vi "MES_Get PLC Address.vi"(0 "StationName":string, 1 "LineNum":string, 5 "Main":string, 9 "VariableName":string, 11 "error in (no error)":errorcluster, 12 "Alarm":bool=TRUE) -> (3 "IPList":string[](array[string]), 4 "Value":T1, 10 "Array":bool[](array[boolean]), 13 "PLC DB DBB2List":string[](array[string]), 14 "PLC DB DBB1List":string[](array[string]), 15 "error out":errorcluster)   [LabVIEW 2021, in "SQLite.lvclass"]
doc: "读取MES与PLC通讯的IP地址，DB块，DBB地址，format\n# 2020-5-13 13:25:16\n# daikinyi\n蒋松\njiangsong@outlook.com"
uses:
  SQLite.lvclass
  Control/PLCAddress value Type.ctl
  SQLiteFileName.ctl
  TabelFullName.ctl
  <userlib>/LabSQL/LabSQL.lvlib
  <userlib>/sushu/sushu.lvlib
panel:
  out "number (0 to 1)":dbl
  out "Select SQL CMD":string
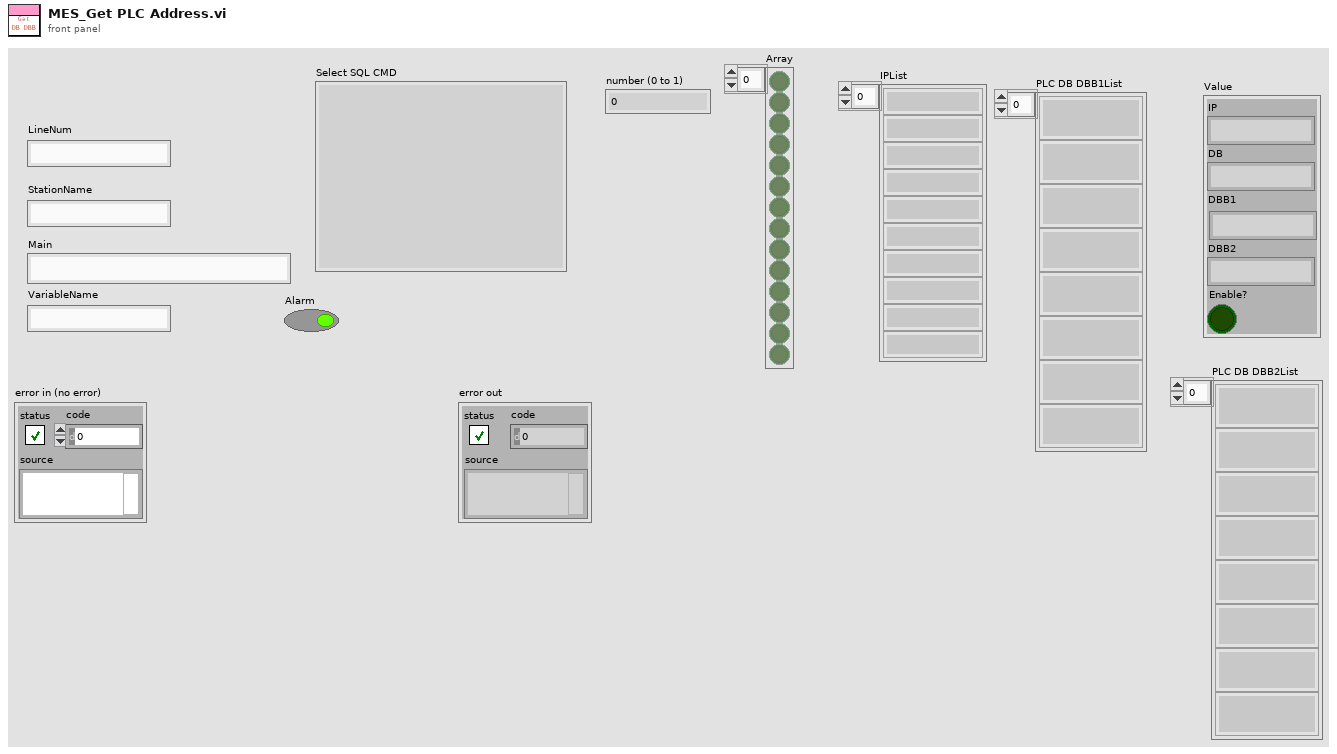
[diagram p1: front panel]
types:
  T1 = typedef "SQLite.lvclass/PLCAddress value Type.ctl" = cluster{"IP":string, "DB":string, "DBB1":string, "DBB2":string, "Enable?":bool}
  T2 = enum16{"Initialize", "Read", "Write", "UnInitialize"}
  T3 = typedef "SQLite.lvclass/TabelFullName.ctl" = string
  T4 = typedef "SQLite.lvclass/SQLiteFileName.ctl" = string
  T5 = cluster{"Current VI Reference":refnum<vi>, "Close Panel on Exit?":bool}
  T6 = cluster{"Core":cluster{"Current VI Reference":refnum<vi>, "Close Panel on Exit?":bool}, "VI Name":string}
  T7 = enum16{"Other", "SQL2008", "SQLite", "Access", "MySQL"}
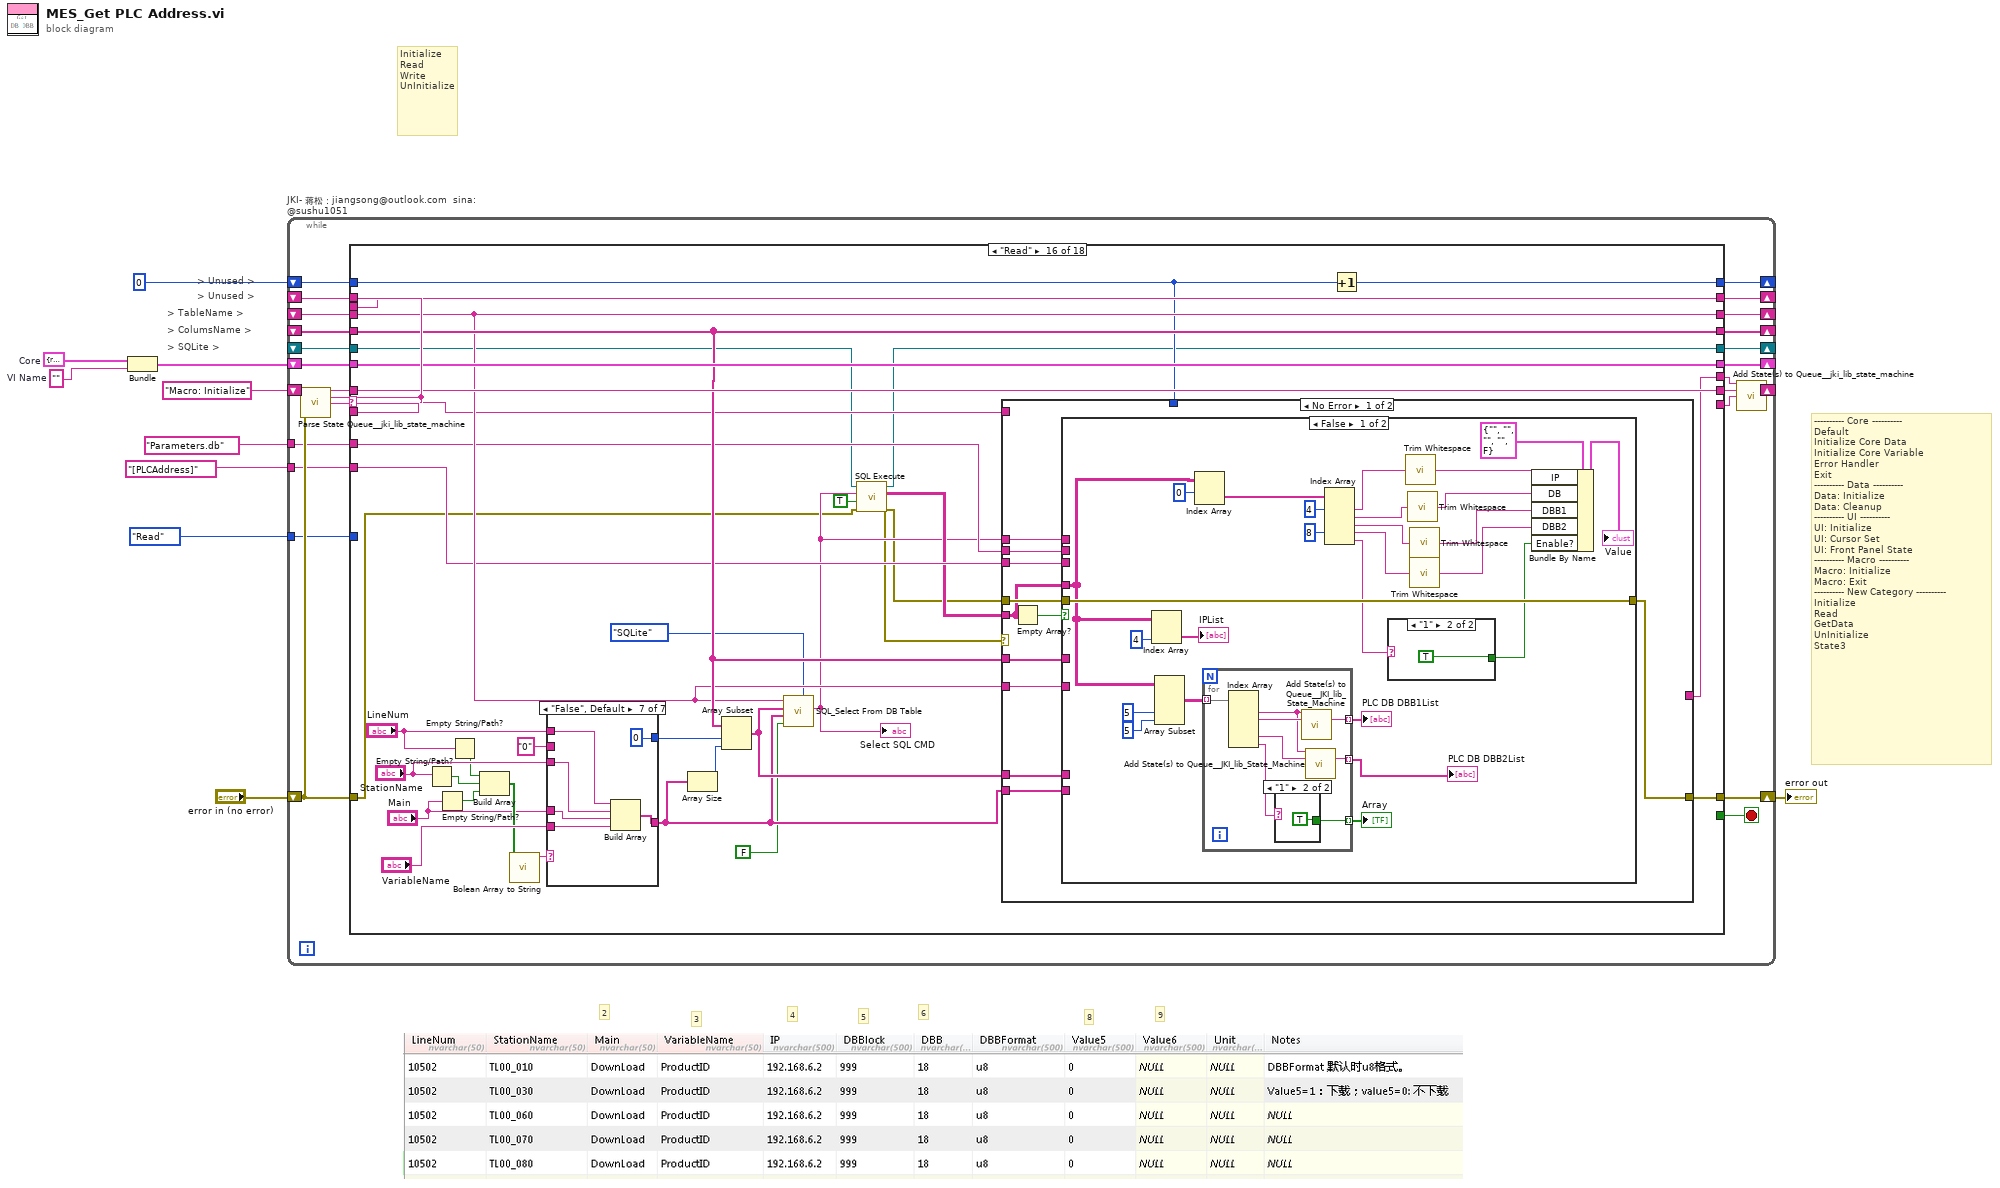
[diagram p0: block diagram]
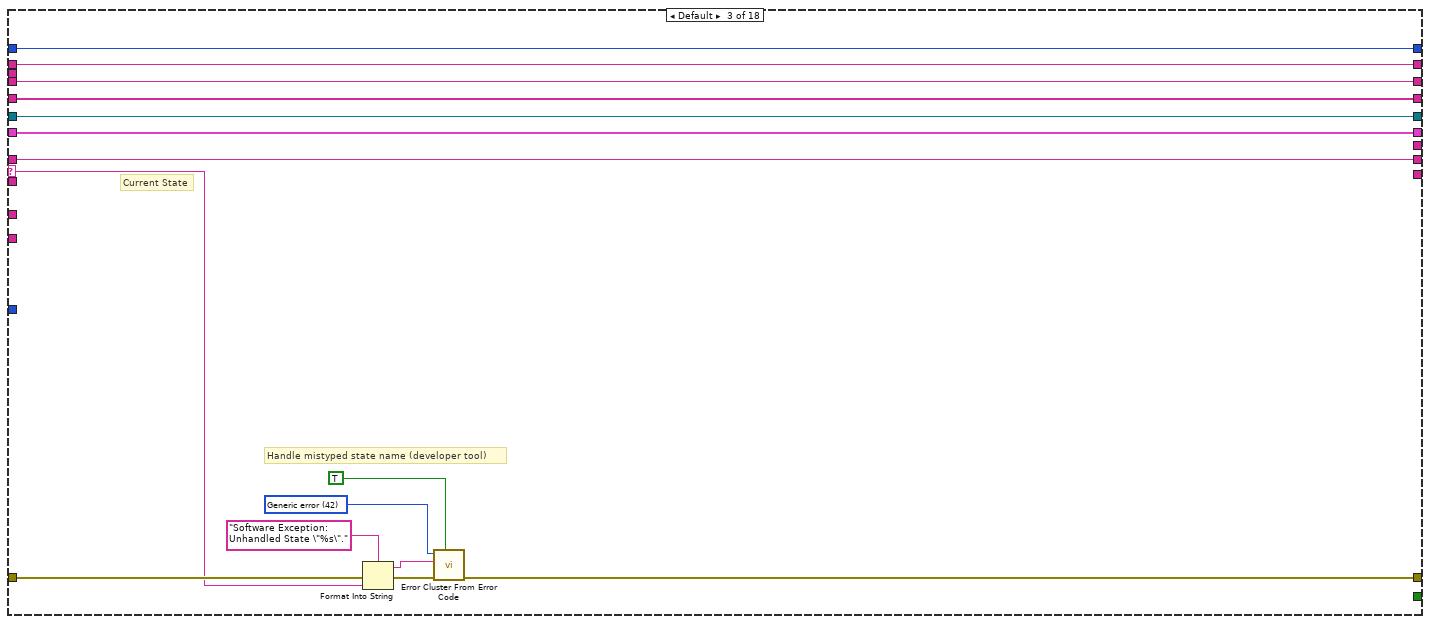
[diagram p4: hidden frame]
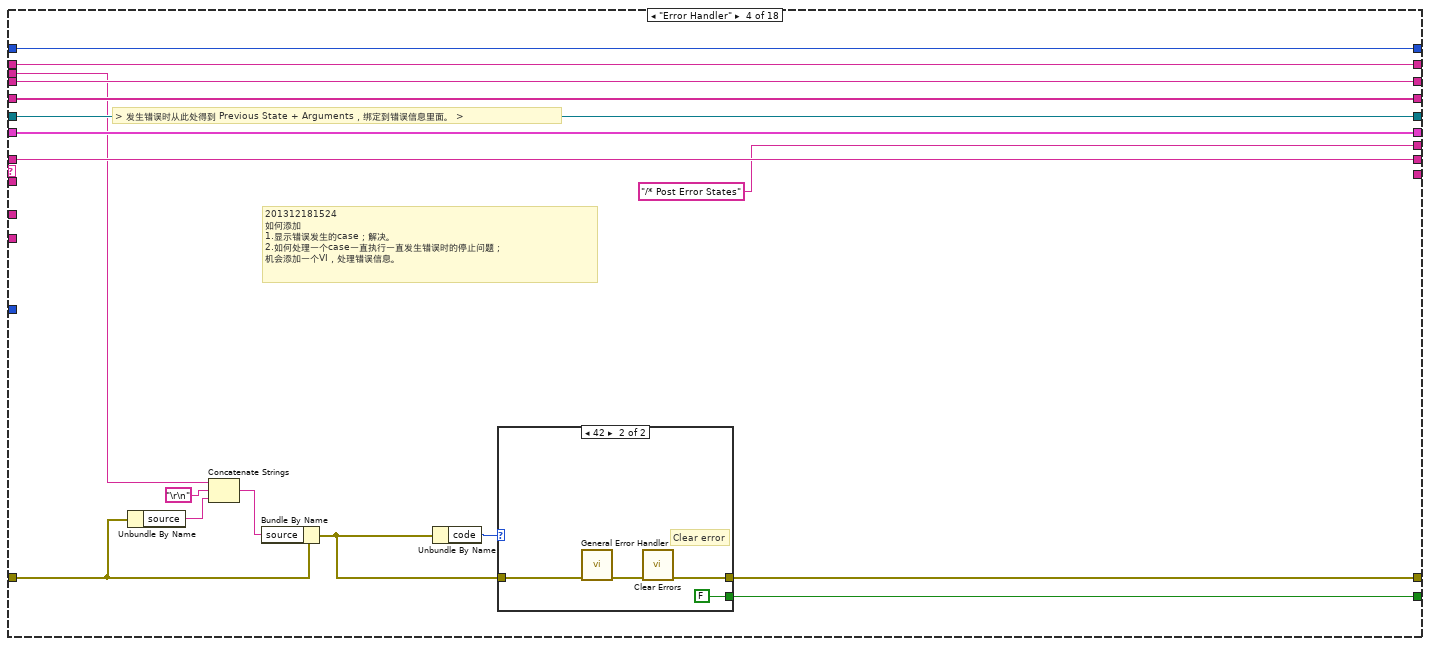
[diagram p5: hidden frame]
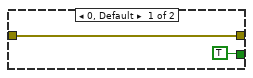
[diagram p6: hidden frame]
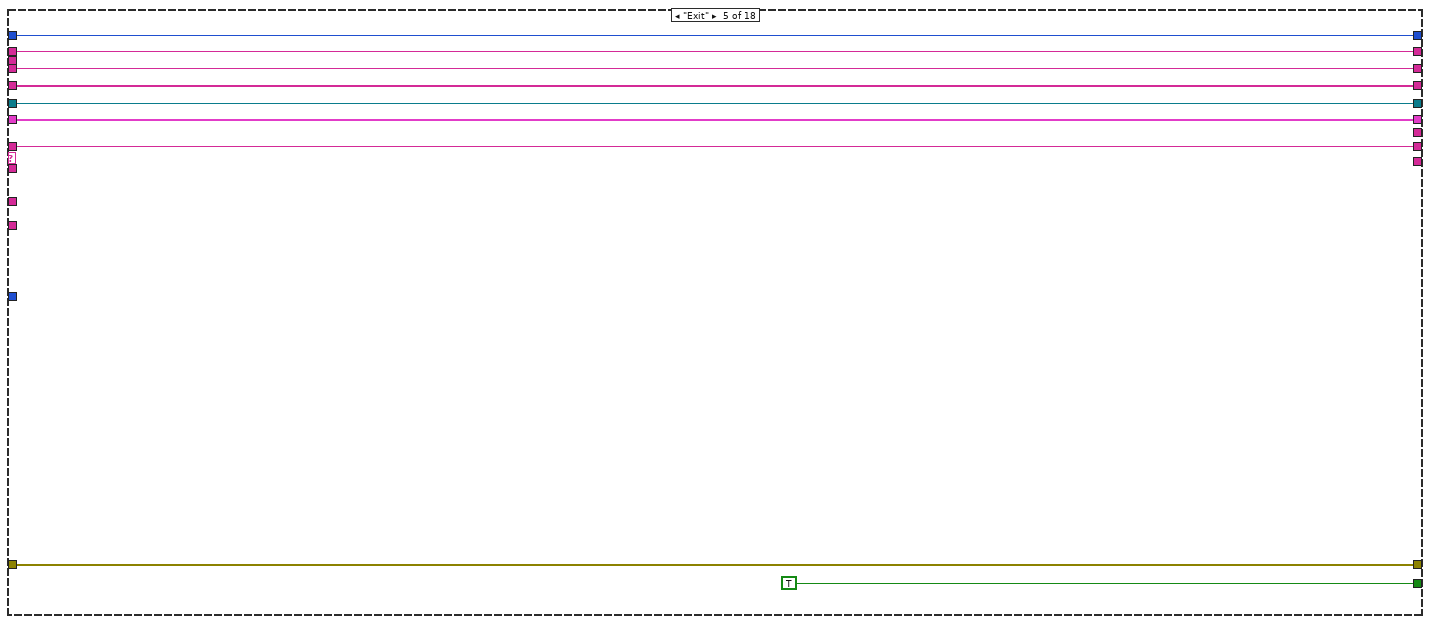
[diagram p7: hidden frame]
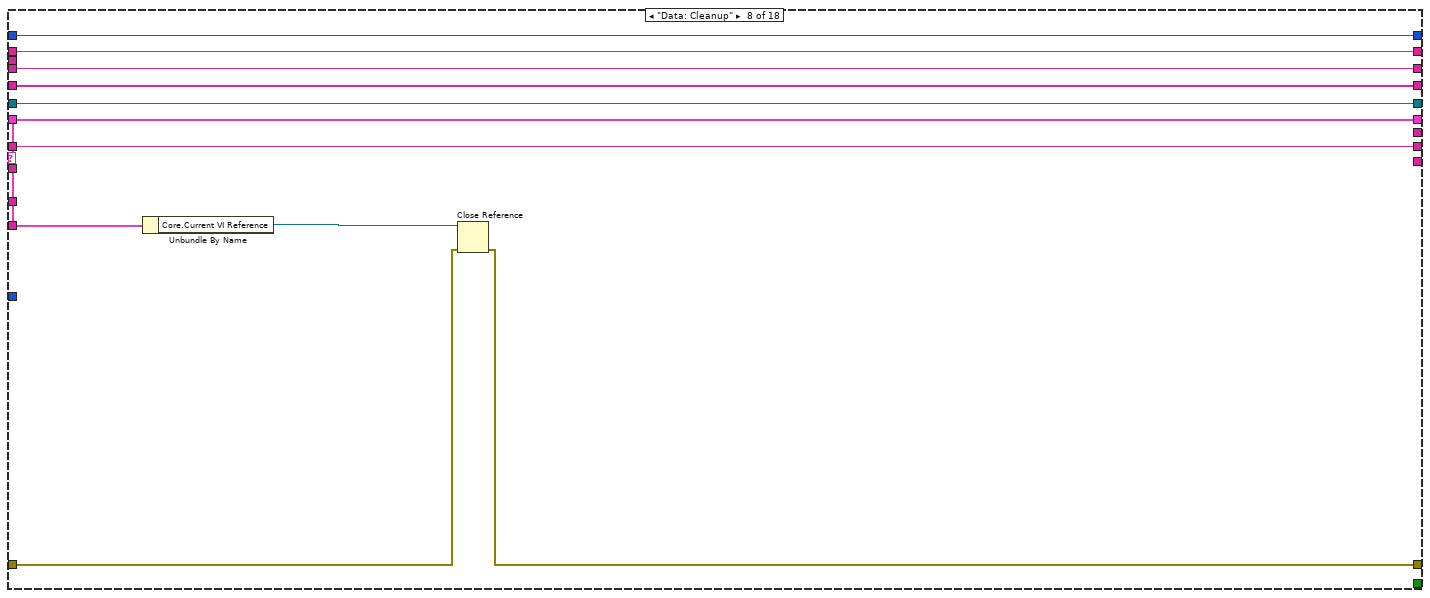
[diagram p10: hidden frame]
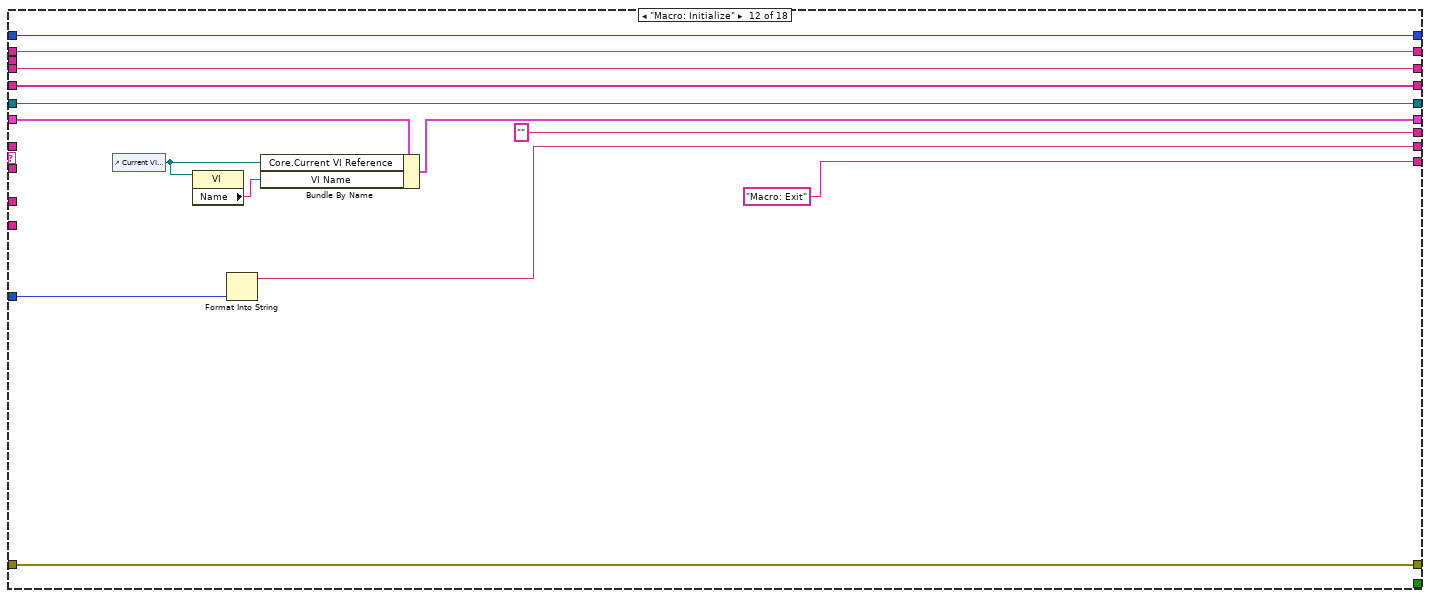
[diagram p14: hidden frame]
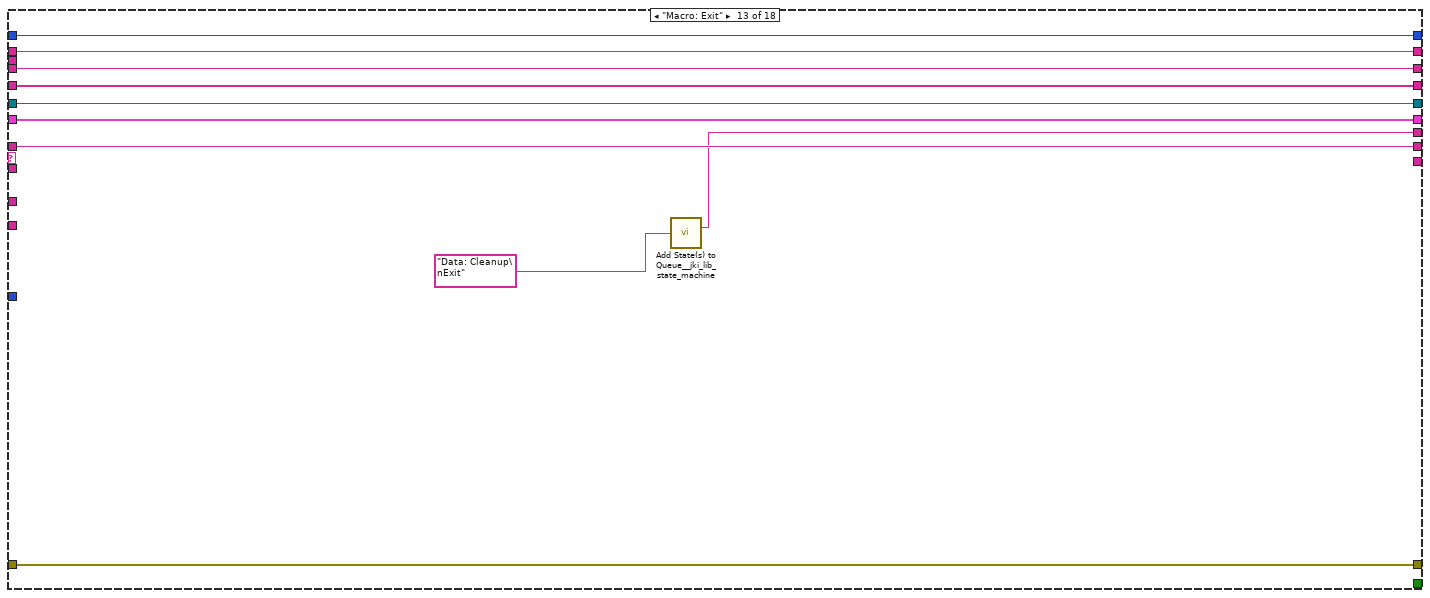
[diagram p15: hidden frame]
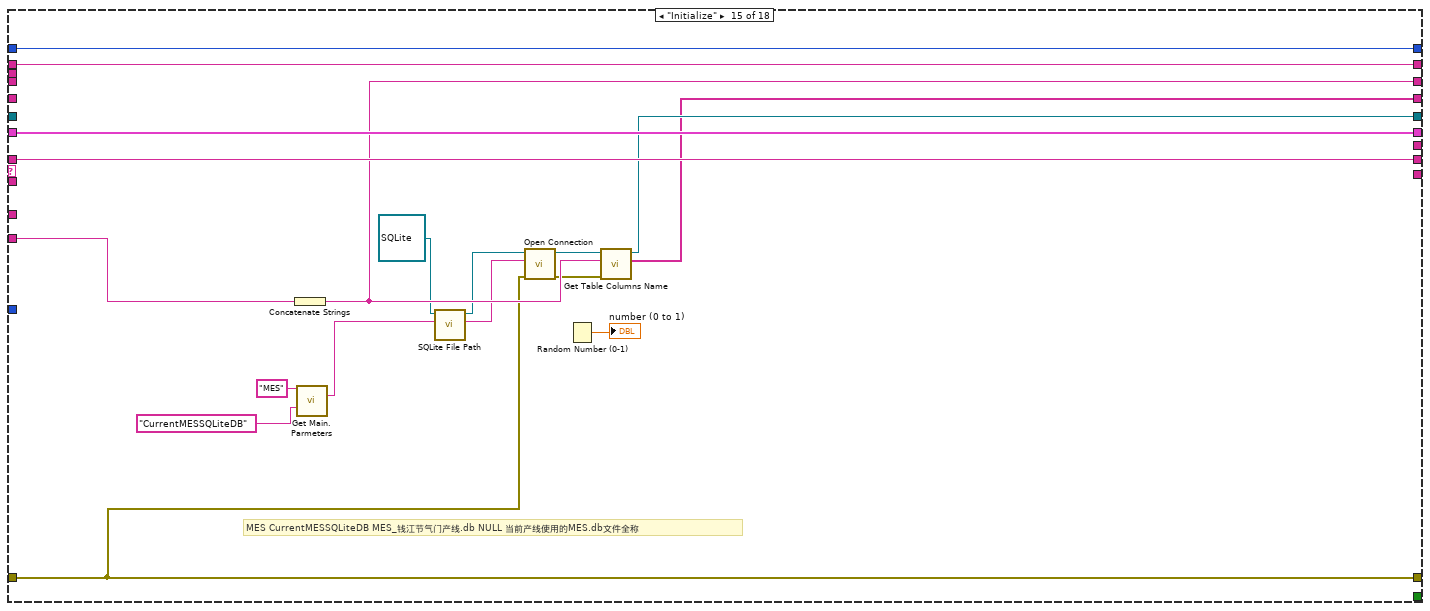
[diagram p17: hidden frame]
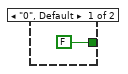
[diagram p18: hidden frame]
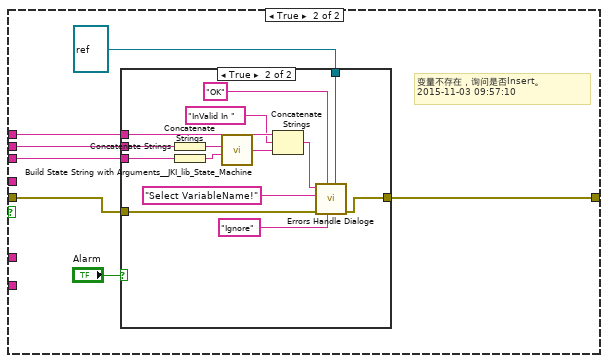
[diagram p20: hidden frame]
diagram:
  w10 = ""  # VI Name
  w9 = T5 {"Current VI Reference"=refnum, "Close Panel on Exit?"=FALSE}  # Core
  # "9"
  # "8"
  # "2"
  # "6"
  # "5"
  # "4"
  # "3"
  # "Initialize\nRead\nWrite\nUnInitialize"
  # "> Unused >"
  # "> SQLite >"
  # "> ColumsName >"
  # "> TableName >"
  # "> Unused >"
  # "---------- Core ----------\nDefault\nInitialize Core Data\nInitialize Core Variable\nError Handler\nExit\n---------- Data ----------\nData: Initialize\nData: Cleanup\n---------- UI ----------\nUI: Initialize\nUI: Cursor Set\nUI: Front Panel State\n---------- Macro ----------\nMacro: Initialize\nMacro: Exit\n---------- New Category ----------\nInitialize\nRead\nGetData\nUnInitialize\nState3"
  n1 = Bundle("Core"=w9, "VI Name"=w10) -> (w8:T6)  [unwired: 1 in]
  n2 = while "JKI- 蒋松：jiangsong@outlook.com  sina: @sushu1051" {
    shift-right: [w34] -> w3
    shift-left: "error in (no error)" -> [w32]
    shift-right: [w22] -> _
    shift-left: "Macro: Initialize" -> [w23]
    shift-right: [w29] -> _
    shift-left: _ -> [w31]
    shift-right: [w30] -> _
    shift-left: _ -> [w11]
    shift-right: [w24] -> _
    shift-left: w8 -> [w27]
    shift-right: [w25] -> _
    shift-left: _ -> [w18]
    shift-right: [w26] -> _
    shift-left: _ -> [w28]
    shift-right: [w17] -> _
    shift-left: 0 -> [w16]
    tunnel: T2."Read" ("CMD") -> [w15]
    tunnel: T4 "Parameters.db" ("SQLiteFileName") -> [w14]
    tunnel: T3 "[PLCAddress]" ("TabelFullName") -> [w13]
    stop <- w33 stop-if-true
    n3 = call <vilib>:"Parse State Queue__jki_lib_state_machine.vi"("State Queue"=w23, "Error In (no error)"=w32) -> ("Remaining States"=w36:string, "Current State"=w12:string, "Arguments"=w35:string)  [unwired: 10 in, 1 out]
    n4 = case shown="\"Read\"" w12 {
      selector: w12 -> [_ _ w55 _ _ _ _ _ _ _ _ _ _ _ _ w220 _ _]
      tunnel: w36 -> [w44 w46 w54 w76 w92 w101 w110 w117 w127 w135 w143 _ w166 w175 w199 w234 w361 w371]
      tunnel: w35 -> [_ _ _ _ _ _ _ _ _ _ _ _ _ _ _ _ _ _]
      tunnel: [w43 w52 w56 w70 w94 w103 w112 w119 w129 w137 w145 w160 w170 w178 w189 w221 w354 w362] -> w34
      tunnel: w32 -> [w43 w52 w57 w80 w94 w103 w112 w120 w129 w137 w145 w160 w170 w178 w189 w213 w354 w363]
      tunnel: [w44 w46 w54 w76 w92 w101 w110 w117 w127 w135 w143 w151 w166 w175 w199 w234 w361 w371] -> w21
      tunnel: [_ _ _ w69 TRUE _ _ _ _ _ _ _ _ _ _ _ _ _] -> w33
      tunnel: w12 -> [w42 w51 w67 w84 w99 w107 w115 w125 w133 w141 w149 w163 w173 w181 w198 w222 w355 w370]
      tunnel: w31 -> [w41 w50 w66 w83 w98 w106 w114 w124 w132 w140 w148 w162 w172 w180 _ w225 w360 w369]
      tunnel: [w42 w51 w67 w84 w99 w107 w115 w125 w133 w141 w149 w163 w173 w181 w198 w222 w355 w370] -> w30
      tunnel: [w41 w50 w66 w83 w98 w106 w114 w124 w132 w140 w148 w162 w172 w180 w191 w225 w360 w369] -> w29
      tunnel: w28 -> [w40 w49 w65 w82 w97 w105 w113 w123 w131 w139 w147 w161 w171 w179 _ w226 w359 w368]
      tunnel: w18 -> [w38 w47 w64 w74 w93 w102 w111 w118 w128 w136 w144 w159 w167 w176 _ w217 w358 w365]
      tunnel: w27 -> [w39 w48 w63 w81 w96 w104 w108 w121 w130 w138 w146 w153 w168 w177 w197 w233 w357 w367]
      tunnel: [w40 w49 w65 w82 w97 w105 w113 w123 w131 w139 w147 w161 w171 w179 w192 w226 w359 w368] -> w26
      tunnel: [w38 w47 w64 w74 w93 w102 w111 w118 w128 w136 w144 w159 w167 w176 w193 w215 w358 w364] -> w25
      tunnel: [w39 w48 w63 w81 w96 w104 w108 w121 w130 w138 w146 w152 w168 w177 w197 w233 w357 w367] -> w24
      tunnel: [_ _ _ "/* Post Error States" _ _ _ _ _ _ _ "" w165 _ _ w219 _ _] -> w20
      tunnel: [_ _ _ _ _ _ _ _ _ _ _ "Macro: Exit" _ _ _ _ _ _] -> w19
      tunnel: w16 -> [w37 w45 w53 w73 w91 w100 w109 w116 w126 w134 w142 w158 w164 w174 w196 w218 w356 w366]
      tunnel: [w37 w45 w53 w73 w91 w100 w109 w116 w126 w134 w142 w158 w164 w174 w196 w232 w356 w366] -> w17
      tunnel: w15 -> [_ _ _ _ _ _ _ _ _ _ _ w150 _ _ _ _ _ _]
      tunnel: w14 -> [_ _ _ _ _ _ _ _ _ _ _ _ _ _ _ w223 _ _]
      tunnel: w13 -> [_ _ _ _ _ _ _ _ _ _ _ _ _ _ w194 w224 _ _]
      tunnel: w11 -> [_ _ _ w68 _ _ _ _ _ _ _ _ _ _ _ _ _ _]
      frame "Idle" {
      }
      frame "---------- Core ----------" {
      }
      frame Default {
        w59 = 42 items=["No error", "Argument error", "Memory is full", "Out of zone", "End of file", "File already open", "Generic file I/O error", "File not found", "File permission error", "Disk is full", "Duplicate path", "Too many files open", "System feature not enabled", "Resource file not found", "Cannot add resource", "Resource not found", "Image not found", "Image memory error", "Pen does not exist", "Config type invalid", "Config token not found", "Config parse error", "Config memory error", "Bad external code format", "Bad external code offset", "External code not present", "Null window", "Destroy window error", "Null menu", "Print aborted", "Bad print record", "Print driver error", "Windows error during printing", "Memory error during printing", "Print dialog error", "Generic print error", "Invalid device refnum", "Device not found", "Device parameter error", "Device unit error", "Cannot open device", "Device call aborted", "Generic error", "Cancelled by user", "Object ID too low", "Object ID too high", "Object not in heap", "Unknown heap", "Unknown object (invalid DefProc)", "Unknown object (DefProc not in table)", "Message out of range", "Invalid (null) method", "Unknown message", "Manager call not supported", "Bad address", "Network operation in progress", "Network operation timed out", "Connection is busy", "Network attribute not supported", "Network error", "Address in use", "System out of memory", "Connection aborted", "Connection refused", "Not connected", "Already connected", "Connection closed", "Initialization error (interapplication manager)", "Bad occurrence", "Wait on unbound occurrence handler", "Occurrence queue overflow", "Datalog type conflict", "Unused", "Unrecognized type (interapplication manager)", "Memory corrupt", "Failed to make temporary DLL", "Old CIN version", "Drag socket not found", "Failed to load drop-object", "Failed to register OLE object", "Failed to release OLE object", "Format specifier type mismatch", "Unknown format specifier", "Too few format specifiers", "Too many format specifiers", "Scan failed", "Newer CIN version", "Error converting to variant", "Runtime menu error", "Password tampered", "Variant attribute not found", "Incompatible variant data type", "Event data is not available", "Event Store is not present", "Occurrence is not found", "Event Queue is not created", "Event info is not available", "Refnum passed is NULL", "Error retrieving Class GUID", "Error retrieving CoClass GUID", "Error retrieving TypeLib GUID.", "Bad built application magic bytes.", "Specific driver is different from the specific driver associated with the Logical Name.", "There is no session opened to the class driver.", "Max Error", "MAX - Error with config objects", "MAX - Error loading configuration", "MAX - Group not supported"]
        # "Current State"
        # "Handle mistyped state name (developer tool)"
        n5 = Format Into String(format string="Software Exception: Unhandled State \"%s\"." ("message"), error in=w57, w55) -> (resulting string=w60:string, error out=w61:errorcluster)  [unwired: 1 in]
        n6 = call <vilib>:"Error Cluster From Error Code.vi"("show call chain? (False)"=TRUE, "error in (no error)"=w61, "error message (\"\")"=w60, "error code (0)"=w59) -> ("error out"=w56:errorcluster)  [unwired: 5 in]
      }
      frame "Error Handler" {
        # "> 发生错误时从此处得到 Previous State + Arguments，绑定到错误信息里面。 >"
        # "201312181524\n如何添加\n1.显示错误发生的case；解决。\n2.如何处理一个case一直执行一直发生错误时的停止问题；\n机会添加一个VI，处理错误信息。"
        # "Clear error"
        n7 = Unbundle By Name(w80) -> ("source"=w78:string)
        n8 = Concatenate Strings(w68, "\r\n", w78) -> (w77:string)
        n9 = Bundle By Name(cluster=w80, "source"=w77) -> (w71:errorcluster)
        n10 = Unbundle By Name(w71) -> ("code"=w72:i32)
        n11 = case shown="42" w72 {
          tunnel: [TRUE FALSE] -> w69
          tunnel: w71 -> [w86 w89]
          tunnel: [w86 w87] -> w70
          frame 0, Default {
          }
          frame 42 {
            n12 = call <vilib>:"General Error Handler.vi"("error in (no error)"=w89) -> ("error out"=w88:errorcluster)  [unwired: 10 in, 4 out]
            n13 = call <vilib>:"Clear Errors.vi"("error in (no error)"=w88) -> ("error out"=w87:errorcluster)  [unwired: 5 in, 1 out]
          }
        }
      }
      frame "Exit" {
      }
      frame "---------- Data ----------" {
      }
      frame "Data: Initialize" {
      }
      frame "Data: Cleanup" {
        n14 = Unbundle By Name(w121) -> ("Core.Current VI Reference"=w122:refnum<vi>)
        n15 = Close Reference(reference=w122, error in (no error)=w120) -> (error out=w119:errorcluster)
      }
      frame "---------- UI ----------" {
      }
      frame "UI: Initialize" {
      }
      frame "---------- Macro ----------" {
      }
      frame "Macro: Initialize" {
        n16 = control-ref of="Current VI Reference"() -> (w154:refnum<vi>)
        n17 = property class="VI"(reference=w154) -> ("Name"=w155:string)  [unwired: 1 in, 2 out]
        n18 = Format Into String(w150) -> (resulting string=w151:string)  [unwired: 3 in, 1 out]
        n19 = Bundle By Name(cluster=w153, "Core.Current VI Reference"=w154, "VI Name"=w155) -> (w152:T6)
      }
      frame "Macro: Exit" {
        n20 = call <vilib>:"Add State(s) to Queue__jki_lib_state_machine.vi"("State(s) at Back (\"\")"="Data: Cleanup\nExit") -> ("States Out"=w165:string)  [unwired: 14 in]
      }
      frame "---------- New Category ----------" {
      }
      frame "Initialize" {
        # "MES\tCurrentMESSQLiteDB\tMES_钱江节气门产线.db\tNULL\t当前产线使用的MES.db文件全称"
        n21 = Concatenate Strings(w194) -> (w191:string)
        n22 = call "Get Main.Parmeters.vi"("Main"="MES", "VariableName"="CurrentMESSQLiteDB" ("Main")) -> ("Value"=w182:string)  [unwired: 6 in, 7 out]
        n23 = call "SQLite File Path.vi"("SQLiteFileName"=w182, "SQLite in"=refnum<class "SQLite.lvclass"> refnum ("SQLite.lvclass")) -> ("string"=w188:string, "SQLite out"=w186:refnum<class "SQLite.lvclass">)  [unwired: 7 in, 1 out]
        n24 = call-dynamic "Open Connection.vi"("error in (no error)"=w189, "ConnectionString"=w188, "HostDB in"=w186) -> ("error out"=w190:errorcluster, "HostDB out"=w195:refnum<class "SQLite.lvclass">)  [unwired: 7 in]
        n25 = Random Number (0-1)() -> (number: 0 to 1=→"number (0 to 1)":dbl)
        n26 = call-dynamic "Get Table Columns Name.vi"("error in (no error)"=w190, "TableName"=w191, "HostDB in"=w195) -> ("Table_ColunmsList"=w192:string[], "HostDB out"=w193:refnum<class "SQLite.lvclass">)  [unwired: 4 in, 3 out]
      }
      frame "Read" {
        n27 = Empty String/Path?(string/path="StationName") -> (empty?=w209:bool)
        n28 = Empty String/Path?(string/path="Main") -> (empty?=w208:bool)
        n29 = Empty String/Path?(string/path="LineNum") -> (empty?=w202:bool)
        n30 = Build Array(w202, w209, w208) -> (w207:bool[])
        n31 = call <userlib>:"Bolean Array to String.vi"("Bolean Array"=w207) -> ("Bolean String"=w206:string)  [unwired: 10 in]
        n32 = case shown="\"False\", Default" w206 {
          tunnel: [w322 w326 w329 w335 w341 w347 w353] -> w229
          tunnel: "Main" -> [w321 w323 _ w332 _ w342 w352]
          tunnel: "VariableName" -> [w320 w325 w328 w334 w340 w346 w351]
          tunnel: "StationName" -> [w318 _ _ _ w337 w343 w350]
          tunnel: [1 ("index") 2 ("index") 3 ("index") 0 ("index") 0 ("index") 0 ("index") 0 ("index")] -> w204
          tunnel: "LineNum" -> [_ _ _ w330 w338 w344 w348]
          tunnel: "0" ("element") -> [_ _ _ w331 w336 _ _]
          frame "100" {
            n33 = Build Array(w318, w321, w320) -> (w322:string[])
          }
          frame "110" {
            n34 = Build Array(w323, w325) -> (w326:string[])
          }
          frame "111" {
            n35 = Build Array(w328) -> (w329:string[])
          }
          frame "010" {
            n36 = Build Array(w330, w331, w332, w334) -> (w335:string[])
          }
          frame "001" {
            n37 = Build Array(w338, w337, w336, w340) -> (w341:string[])
          }
          frame "000" {
            n38 = Build Array(w344, w343, w342, w346) -> (w347:string[])
          }
          frame "False", Default {
            n39 = Build Array(w348, w350, w352, w351) -> (w353:string[])
          }
        }
        n40 = Array Size(array=w229) -> (size(s)=w228:i32)
        n41 = Array Subset(array=w226, index=w204, length=w228) -> (w231:string[])
        n42 = call <userlib>:"SQL_Select From DB Table.vi"("DB Type"=T7."SQLite", "Check ASCII?"=FALSE, "ColumnsValue"=w229, "ColumnsNameList"=w231, "TableName"=w225) -> ("Select SQL CMD"=w214:string)  [unwired: 6 in]
        "Select SQL CMD" <- w214
        n43 = call-dynamic "SQL Execute.vi"("error in (no error)"=w213, "Return Data (T)"=TRUE, "Command Text"=w214, "HostDB in"=w217) -> ("error out"=w212:errorcluster, "Table Control"=w216:string[][], "HostDB out"=w215:refnum<class "SQLite.lvclass">)  [unwired: 3 in, 2 out]
        n44 = case shown="No Error" w212 {
          selector: w212 -> [_ w310]
          tunnel: w231 -> [w245 _]
          tunnel: w212 -> [w244 w317]
          tunnel: w214 -> [w242 _]
          tunnel: w216 -> [w241 _]
          tunnel: w229 -> [w240 _]
          tunnel: w226 -> [w239 _]
          tunnel: w225 -> [w238 _]
          tunnel: w224 -> [w237 _]
          tunnel: w223 -> [w236 _]
          tunnel: [w235 w316] -> w221
          tunnel: w220 -> [_ w309]
          tunnel: [_ w308] -> w219
          tunnel: w218 -> [_ w307]
          frame No Error {
            n45 = Empty Array?(array=w241) -> (empty?=w243:bool)
            n46 = case shown="False" w243 {
              tunnel: [w271 w289] -> w235
              tunnel: w239 -> [_ _]
              tunnel: w238 -> [_ _]
              tunnel: w240 -> [_ _]
              tunnel: w245 -> [_ _]
              tunnel: w244 -> [w271 w290]
              tunnel: w242 -> [_ w286]
              tunnel: w236 -> [_ w288]
              tunnel: w237 -> [_ w287]
              tunnel: w241 -> [w261 _]
              frame False {
                n47 = Index Array(array=w261, index (col)=4 ("disabled index (col)")) -> (element=→"IPList":string[])  [unwired: 1 in]
                n48 = Array Subset(array=w261, index (col)=5 ("index"), length (col)=5 ("length")) -> (w258:string[][])  [unwired: 2 in]
                n49 = Index Array(array=w261, index (row)=0) -> (element=w269:string[])  [unwired: 1 in]
                n50 = for {
                  tunnel: w258 -> [w281] mode=indexing
                  tunnel: [w279] -> w257 mode=indexing
                  tunnel: [w277] -> w247 mode=indexing
                  tunnel: [w274] -> w246 mode=indexing
                  n51 = Index Array(array=w281) -> (element #1=w278:string, element #2=w280:string, element #4=w276:string, element #5=w275:string)  [unwired: 5 in, 1 out]
                  n52 = case shown="\"1\"" w275 {
                    tunnel: [FALSE ("Boolean") TRUE ("Boolean")] -> w274
                    frame "0", Default {
                    }
                    frame "1" {
                    }
                  }
                  n53 = call <vilib>:"Add State(s) to Queue__JKI_lib_State_Machine.vi"("State(s) in Front (\"\")"=w278, "State(s) in (\"\")"=w280) -> ("States Out"=w279:string)  [unwired: 13 in]
                  n54 = call <vilib>:"Add State(s) to Queue__JKI_lib_State_Machine.vi"("State(s) in Front (\"\")"=w278, "State(s) in (\"\")"=w276) -> ("States Out"=w277:string)  [unwired: 13 in]
                }
                "PLC DB DBB1List" <- w257
                "PLC DB DBB2List" <- w247
                "Array" <- w246
                n55 = Index Array(array=w269, index #1=4 ("index"), index #4=8 ("index")) -> (element #1=w267:string, element #2=w266:string, element #3=w265:string, element #4=w264:string, element #5=w249:string)  [unwired: 3 in]
                n56 = case shown="\"1\"" w249 {
                  tunnel: [FALSE ("Boolean") TRUE ("Boolean")] -> w248
                  frame "0", Default {
                  }
                  frame "1" {
                  }
                }
                n57 = call <vilib>:"Trim Whitespace.vi"("string"=w267) -> ("trimmed string"=w254:string)  [unwired: 1 in]
                n58 = call <vilib>:"Trim Whitespace.vi"("string"=w266) -> ("trimmed string"=w253:string)  [unwired: 1 in]
                n59 = call <vilib>:"Trim Whitespace.vi"("string"=w265) -> ("trimmed string"=w252:string)  [unwired: 1 in]
                n60 = call <vilib>:"Trim Whitespace.vi"("string"=w264) -> ("trimmed string"=w251:string)  [unwired: 1 in]
                n61 = Bundle By Name(cluster=T1 {"IP"="", "DB"="", "DBB1"="", "DBB2"="", "Enable?"=FALSE} ("Value"), "IP"=w254, "DB"=w253, "DBB1"=w252, "DBB2"=w251, "Enable?"=w248) -> (→"Value":T1)
              }
              frame True {
                # "变量不存在，询问是否Insert。\n2015-11-03 09:57:10"
                n62 = case shown="True" "Alarm" {
                  tunnel: w290 -> [w291 w305]
                  tunnel: [w291 w304] -> w289
                  tunnel: w288 -> [_ w303]
                  tunnel: w287 -> [_ w302]
                  tunnel: w286 -> [_ w301]
                  tunnel: refnum<vi> refnum ("VI Ref") -> [_ w292]
                  frame False {
                  }
                  frame True {
                    n63 = Concatenate Strings(w303) -> (w300:string)
                    n64 = Concatenate Strings(w302) -> (w299:string)
                    n65 = call <vilib>:"Build State String with Arguments__JKI_lib_State_Machine.vi"("Arguments (\"\")"=w299, "State"=w300) -> ("State with Arguments"=w297:string)  [unwired: 4 in]
                    n66 = Concatenate Strings(w301, "InValid In " ("Message"), w297) -> (w296:string)
                    n67 = call <userlib>:"Errors Handle Dialoge.vi"("VI Ref"=w292, "Cancel Text"="Ignore", "OK Text"="OK", "error in (no error)"=w305, "Title Text"="Select VariableName!", "Message"=w296) -> ("error out"=w304:errorcluster)  [unwired: 4 in, 1 out]
                  }
                }
              }
            }
          }
          frame Error {
            n68 = call <vilib>:"Clear Errors.vi"("error in (no error)"=w317) -> ("error out"=w316:errorcluster)  [unwired: 5 in, 1 out]
            n69 = Unbundle By Name(w310) -> ("status"=w306:bool)
            n70 = Equal To 0?(x=w307) -> (x = 0?=w314:bool)
            n71 = And(x=w306, y=w314) -> (x .and. y?=w313:bool)
            n72 = call <vilib>:"Add State(s) to Queue__jki_lib_state_machine.vi"("State(s) in Front (\"\")"="Initialize" ("Remaining States"), "State(s) in (\"\")"=w309) -> ("States Out"=w311:string)  [unwired: 13 in]
            n73 = Select(t=w311, s=w313, f="GetData") -> (s? t:f=w308:string)
          }
        }
        n74 = Increment(x=w218) -> (x+1=w232:i32)
      }
      frame "GetData" {
      }
      frame "UnInitialize" {
        n75 = call-dynamic "Close Connection.vi"("error in (no error)"=w363, "HostDB in"=w365) -> ("error out"=w362:errorcluster, "HostDB out"=w364:refnum<class "SQLite.lvclass">)  [unwired: 8 in]
      }
    }
    n76 = call <vilib>:"Add State(s) to Queue__jki_lib_state_machine.vi"("State(s) in Front (\"\")"=w20, "State(s) in (\"\")"=w21, "State(s) at Back (\"\")"=w19) -> ("States Out"=w22:string)  [unwired: 12 in]
  }
  "error out" <- w3
